vi "FTWLib-Socket-LibraryFilepath.vi"(8 "error in":errorcluster) -> (0 "error out":errorcluster, 1 "Library Version":string, 2 "Library Filepath":path)   [LabVIEW 2013]
uses:
  src/core/error/FTW-ERR-ThrowError.vi
  src/core/error/FTW-ERR-NoErrorConstant.vi
  src/core/string/FTW-STR-ReplaceWhitespace.vi
  src/core/error/FTW-ERR-CallChain.vi
  FTWLib-nanomsg32.dll
  FTWLib-nanomsg64.dll
  FTWLib-nanomsg32.so
panel:
  # "Inputs"
  # "Outputs"
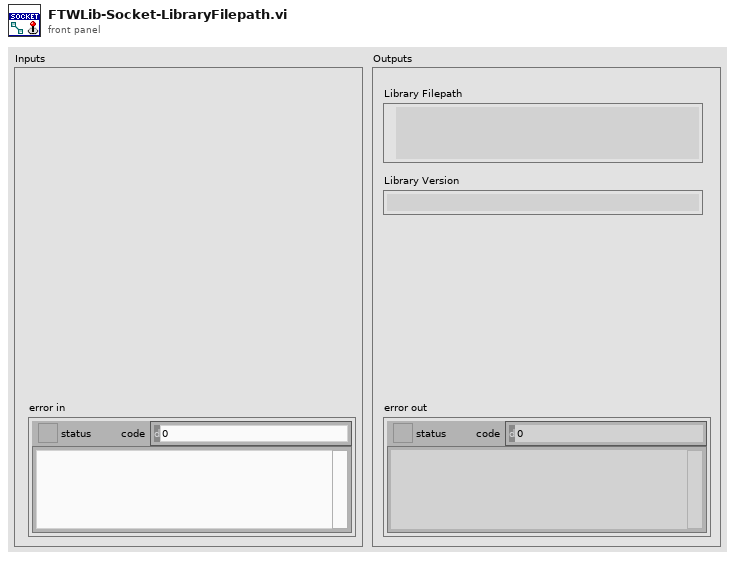
[diagram p1: front panel]
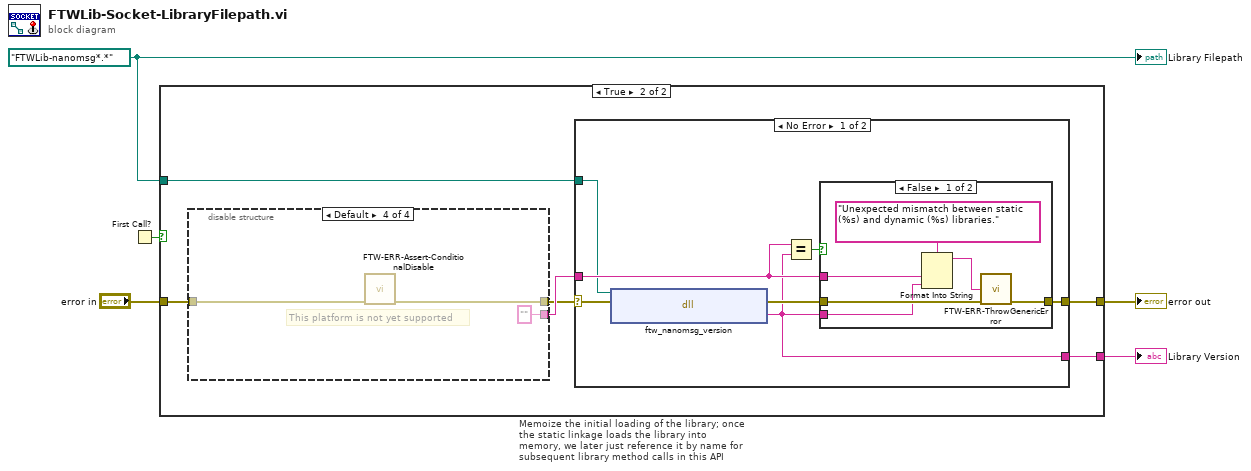
[diagram p0: block diagram]
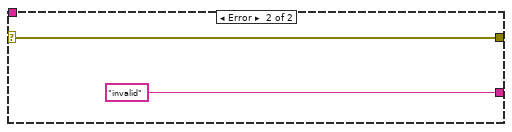
[diagram p4: hidden frame]
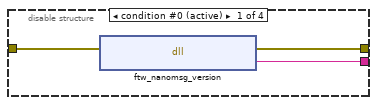
[diagram p5: hidden frame]
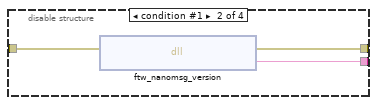
[diagram p6: hidden frame]
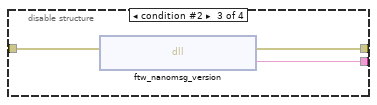
[diagram p7: hidden frame]
diagram:
  w2 = path "FTWLib-nanomsg*.*" ("nanomsg Library Filepath")
  n1 = First Call?() -> (First Call?: T/F=w1:bool)
  n2 = case "Memoize the initial loading of the library; once the static linkage loads the library into memory, we later just reference it by name for subsequent library method calls in this API" shown="True" w1 {
    tunnel: "error in" -> [w6 w10]
    tunnel: [_ w11] -> w3
    tunnel: [w6 w12] -> w4
    tunnel: w2 -> [_ w9]
    frame False {
    }
    frame True {
      n3 = disable-structure shown="Default" {
        disable-tunnel: [w29 w32 w35 "" ("FTW-nanomsg Version")] -> w8
        disable-tunnel: [w30 w33 w36 w39] -> w7
        disable-tunnel: w10 -> [w31 w34 w37 w40]
        frame condition #0 (active) {
          n4 = dll-call lib="C:/Users/Jack/repo/ftw-master/ftw/lib/nanomsg/FTWLib-nanomsg32.dll" fn="ftw_nanomsg_version" label="FTWLib-nanomsg32.dll"(error in=w31) -> (error out=w30:errorcluster, "FTW-nanomsg Version"=w29:string)  [unwired: 2 in, 1 out]
        }
        frame condition #1 {
          n5 = dll-call lib="C:/Users/Jack/repo/ftw-master/ftw/lib/nanomsg/FTWLib-nanomsg64.dll" fn="ftw_nanomsg_version" label="FTWLib-nanomsg64.dll"(error in=w34) -> (error out=w33:errorcluster, "FTW-nanomsg Version"=w32:string)  [unwired: 2 in, 1 out]
        }
        frame condition #2 {
          n6 = dll-call lib="C:/Users/Jack/repo/ftw-master/ftw/lib/nanomsg/FTWLib-nanomsg32.so" fn="ftw_nanomsg_version" label="FTWLib-nanomsg32.so"(error in=w37) -> (error out=w36:errorcluster, "FTW-nanomsg Version"=w35:string)  [unwired: 2 in, 1 out]
        }
        frame condition #3 {
          # "This platform is not yet supported"
          n7 = call "FTW-ERR-Assert-ConditionalDisable.vi"("error in"=w40) -> ("error out"=w39:errorcluster)  [unwired: 14 in]
        }
      }
      n8 = case shown="No Error" w7 {
        selector: w7 -> [w19 w27]
        tunnel: [w16 w27] -> w12
        tunnel: [w14 "invalid" ("Version (minus Build)")] -> w11
        tunnel: w9 -> [w13 _]
        tunnel: w8 -> [w15 _]
        frame No Error {
          n9 = dll-call lib="?" fn="ftw_nanomsg_version"(path in=w13, error in=w19) -> (error out=w17:errorcluster, "FTW-nanomsg Version"=w14:string)  [unwired: 1 in, 1 out]
          n10 = Equal?(x=w15, y=w14) -> (x = y?=w18:bool)
          n11 = case shown="False" w18 {
            tunnel: w17 -> [w25 w26]
            tunnel: [w24 w26] -> w16
            tunnel: w15 -> [w22 _]
            tunnel: w14 -> [w21 _]
            frame False {
              n12 = Format Into String(format string="Unexpected mismatch between static (%s) and dynamic (%s) libraries.", w22, w21) -> (resulting string=w20:string)  [unwired: 2 in, 1 out]
              n13 = call "FTW-ERR-ThrowGenericError.vi"("Error Message"=w20, "error in"=w25) -> ("error out"=w24:errorcluster)  [unwired: 13 in]
            }
            frame True {
            }
          }
        }
        frame Error {
        }
      }
    }
  }
  "error out" <- w4
  "Library Version" <- w3
  "Library Filepath" <- w2
